vi "Read Flange 1 Width.vi"(8 "error in (no error)":errorcluster, 11 "MultiSegmentPipe.lvclass in":refnum<class "MultiSegmentPipe.lvclass">) -> (0 "error out":errorcluster, 2 "Flange1Width":u32, 3 "MultiSegmentPipe.lvclass out":refnum<class "MultiSegmentPipe.lvclass">)   [LabVIEW 2015, in "MultiSegmentPipe.lvclass"]
uses:
  MultiSegmentPipe.lvclass
  MultiSegmentPipe.lvclass/MultiSegmentPipe.ctl
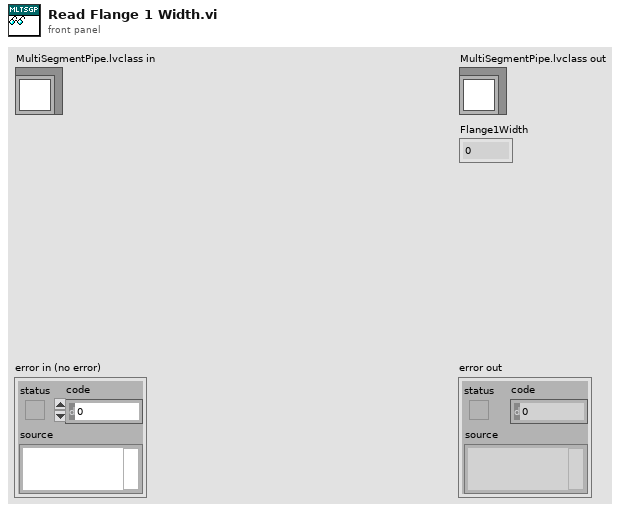
[diagram p1: front panel]
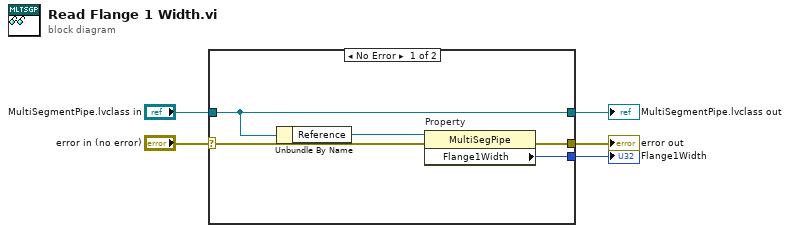
[diagram p0: block diagram]
diagram:
  n1 = case shown="No Error" "error in (no error)" {
    selector: "error in (no error)" -> [w6 w12]
    tunnel: [w9 w12] -> w4
    tunnel: [w8 w11] -> w2
    tunnel: "MultiSegmentPipe.lvclass in" -> [w8 w11]
    tunnel: [w10 _] -> w1
    frame No Error {
      n2 = Unbundle By Name(w8) -> ("Reference"=w7:refnum<vi>)
      n3 = property on="Property" class="MultiSegPipe"(reference=w7, error in=w6) -> (error out=w9:errorcluster, "Flange1Width"=w10:u32)  [unwired: 1 out]
    }
    frame Error {
    }
  }
  "error out" <- w4
  "MultiSegmentPipe.lvclass out" <- w2
  "Flange1Width" <- w1
